vi "Obtain Request Events.vi"(8 "error in":errorcluster, 10 "Create New? (F)":bool) -> (0 "error out":errorcluster, 2 "Data Log Request Events":T1)   [LabVIEW 2025, in "Data Log.lvlib"]
doc: "This VI Obtains/Creates the Requests events that will be used for other modules to communicate with the module that owns this VI. These Requests events will be accessed only via Public API methods for this module.\n\n<b>NOTE</b>: The contents of this VI are automatically generated and modified by the <b>Tools > DQMH Consortium > DQMH</b> utilities. Consider using those utilities instead of making your own modifications to this VI.\n_____\nBased on DQMH Dev Tools: Project Template 7.1.2.1547."
uses:
  Data Log.lvlib
  Request Events--cluster.ctl
  Stop Argument--cluster.ctl
  Show Panel Argument--cluster.ctl
  Hide Panel Argument--cluster.ctl
  Show Diagram Argument--cluster.ctl
  Get Module Execution Status Argument--cluster.ctl
panel:
  # "NOTE: The contents of this VI are automatically generated and modified by the Tools > DQMH Consortium > DQMH utilities. Consider using those utilities instead of making your own modifications to this VI."
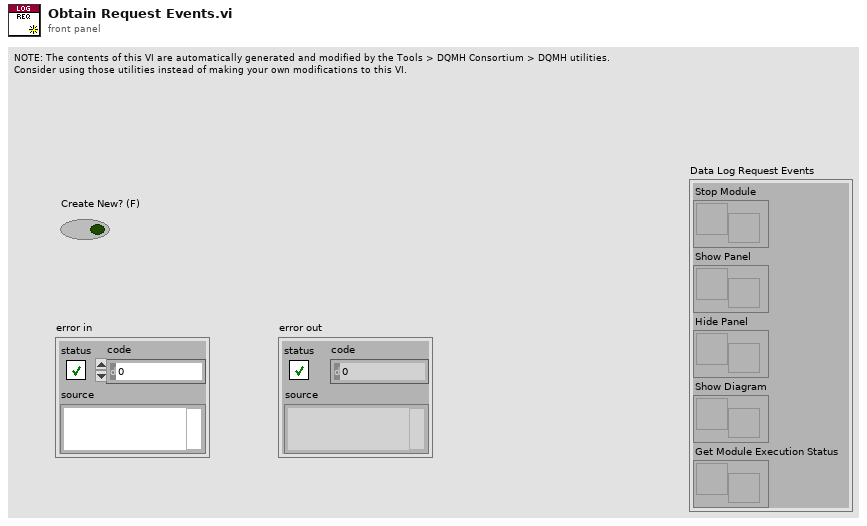
[diagram p1: front panel]
types:
  T1 = typedef "Data Log.lvlib/Request Events--cluster.ctl" = cluster{"Stop Module":refnum<user-event>, "Show Panel":refnum<user-event>, "Hide Panel":refnum<user-event>, "Show Diagram":refnum<user-event>, "Get Module Execution Status":refnum<user-event>}
  T2 = typedef "Data Log.lvlib/Get Module Execution Status Argument--cluster.ctl" = cluster{"Module ID":i32, "Running?":bool}
  T3 = typedef "Data Log.lvlib/Show Diagram Argument--cluster.ctl" = cluster{"Module ID":i32, "Debug?":bool}
  T4 = typedef "Data Log.lvlib/Show Panel Argument--cluster.ctl" = cluster{"Module ID":i32, "Show Panel?":bool}
  T5 = typedef "Data Log.lvlib/Hide Panel Argument--cluster.ctl" = cluster{"Module ID":i32, "Hide Panel?":bool}
  T6 = typedef "Data Log.lvlib/Stop Argument--cluster.ctl" = cluster{"Module ID":i32, "Origin":string, "Exit via Stop Module Req?":bool, "Wait for Module to stop?":bool}
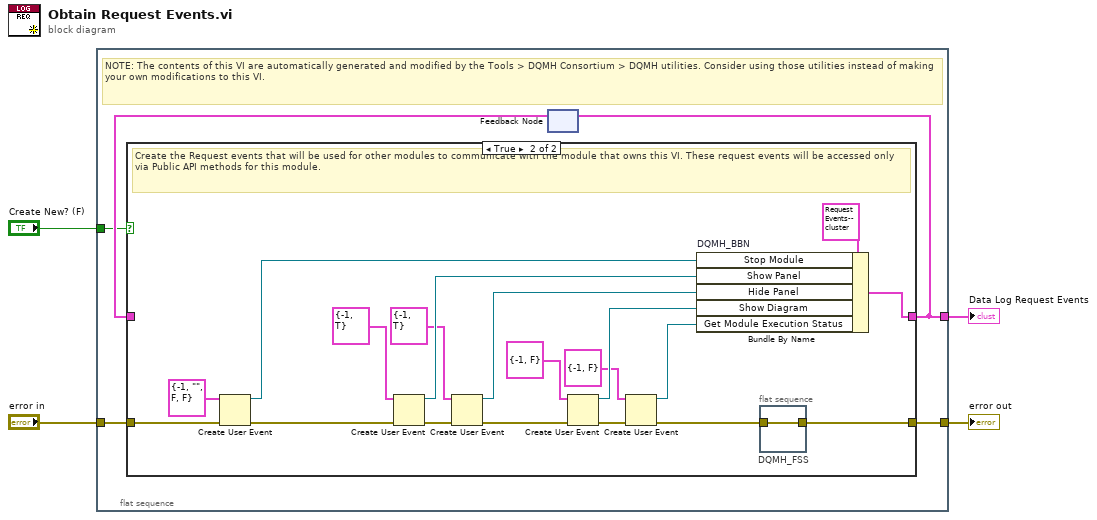
[diagram p0: block diagram]
diagram:
  n1 = flat-sequence {
    tunnel: [w9] -> w4
    tunnel: "error in" -> [w8]
    tunnel: [w6] -> w2
    tunnel: "Create New? (F)" -> [w5]
    frame #0 {
      # "NOTE: The contents of this VI are automatically generated and modified by the Tools > DQMH Consortium > DQMH utilities. Consider using those utilities instead of making your own modifications to this VI."
      n2 = feedback #1() -> (w7:T1)  [unwired: 1 in]
      n3 = case shown="True" w5 {
        tunnel: [w10 w18] -> w9
        tunnel: w8 -> [w10 w30]
        tunnel: [w11 w27] -> w6
        tunnel: w7 -> [w11 _]
        frame False {
        }
        frame True {
          # "Create the Request events that will be used for other modules to communicate with the module that owns this VI. These request events will be accessed only via Public API methods for this module."
          n4 = Create User Event(user event datatype=T6 {"Module ID"=-1, "Origin"="", "Exit via Stop Module Req?"=FALSE, "Wait for Module to stop?"=FALSE} ("Stop Argument"), error in=w30) -> (user event=w28:refnum<user-event>, error out=w25:errorcluster)
          n5 = Create User Event(user event datatype=T4 {"Module ID"=-1, "Show Panel?"=TRUE} ("Show Panel Argument"), error in=w25) -> (user event=w24:refnum<user-event>, error out=w22:errorcluster)
          n6 = Create User Event(user event datatype=T5 {"Module ID"=-1, "Hide Panel?"=TRUE} ("Hide Panel"), error in=w22) -> (user event=w21:refnum<user-event>, error out=w20:errorcluster)
          n7 = Create User Event(user event datatype=T3 {"Module ID"=-1, "Debug?"=FALSE} ("Show Diagram Argument"), error in=w20) -> (user event=w16:refnum<user-event>, error out=w17:errorcluster)
          n8 = Create User Event(user event datatype=T2 {"Module ID"=-1, "Running?"=FALSE} ("Get Module Execution Status Argument"), error in=w17) -> (user event=w13:refnum<user-event>, error out=w14:errorcluster)
          n9 = Bundle By Name "DQMH_BBN"(cluster=T1 {"Stop Module"=refnum, "Show Panel"=refnum, "Hide Panel"=refnum, "Show Diagram"=refnum, "Get Module Execution Status"=refnum} ("output cluster"), "Stop Module"=w28, "Show Panel"=w24, "Hide Panel"=w21, "Show Diagram"=w16, "Get Module Execution Status"=w13) -> (w27:T1)
          n10 = flat-sequence "DQMH_FSS" {
            tunnel: w14 -> [w31]
            tunnel: [w31] -> w18
            frame #0 {
            }
          }
        }
      }
      n11 = feedback-in #1(w6) -> ()
    }
  }
  "Data Log Request Events" <- w2
  "error out" <- w4
